vi "Package.vi"   [LabVIEW 2018, in "Scripts.lvlib"]
uses:
  Scripts.lvlib
  <vilib>/Field R&D Services/Labricator/Toolkit/Type Definitions/LabVIEW Versions.ctl
  <vilib>/Field R&D Services/Labricator/Toolkit/Field_RnD_Services_Labricator_Toolkit.lvlib
panel:
  # "Overview: Builds a VI Package (vip) for LabVIEW versions >= 2015\nRequirements: LabVIEW 2015, VIPM Pro, VIPM API, Labricator Development Kit, Labricator Run-Time\nInstructions: Run this VI.\n\nThis VI attempts to automate the building the VIP file for this add-on as much as possible. If VIPM Pro is not available, then the VIPM API will not work, and the building of the package must be done manually. This VI automates the following manual steps:\n\n1. Save the current project for LabVIEW 2015\n    a. From the Project Explorer window, select File>>Save for Previous Version... A new dialog will appear.\n    b. Select 15.0 from the drop down menu.\n    c. Click Save.... A new dialog will appear. Create a \"target\\15.0\" folder hierarchy in the root project folder (same location as the project file,    \n        .lvproj) if it does not already exist.\n    d. Click OK. All of the contents of the project will be saved to LabVIEW 2015.\n2. Copy the Help source to the target output\n    a. Start Windows Explorer.\n    b. Navigate to the \"<project root>\\src\" folder in Windows Explorer.\n    c. Copy the \"Help\" folder to the \"target\\15.0\\src\" location.\n3. Start LabVIEW 2015 and open the \"target\\15.0\\LIBSSH2.lvproj\" file created in Step 1. Do NOT open any file in the \"target\\15.0\" folder in any other \n    version of LabVIEW.\n4. Build all Source Distributions defined under \"Build Specifications\" tree item in the Project Explorer. A new \"target\\15.0\\builds\" folder will be \n    created with a sub-folder for each component.\n5. Expand the \"Configurations\" virtual folder in the Project Explorer and double click on the \"LabPack.vipb\" file. This will start the VIPM application.\n6. Click the \"Build\" icon near the top of the window for the LabPack package specification. Do NOT alter any values, but ensure \"2015\" is selected at \n    the top right.\n7. Once the package is built, it will be available at \"target\\15.0\\packages\".\n\nNote, any version newer than LabVIEW 2015 can be used to run this VI and still have the package built for LabVIEW 2015, but the LabVIEW 2015 development environment must be installed.\n\nWhen this VI runs, it will automatically start LabVIEW 2015, build all of the components, start VIPM, build the package, then close both LabVIEW 2015 and VIPM. Another VI, \"Build Target.vi\" will run during this process. Do not abort or close this VI while running."
types:
  T1 = typedef "Field_RnD_Services_Labricator_Toolkit.lvlib/LabVIEW Versions.ctl" = enum16{"2009", "2010", "2011", "2012", "2013", "2014", "2015", "2016", "2017", "2018"}
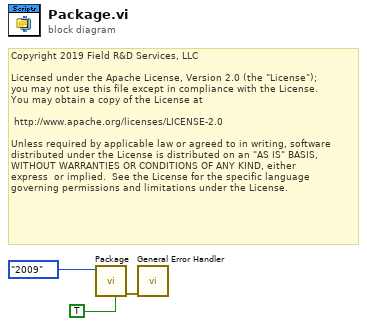
[diagram p0: block diagram]
diagram:
  # "Copyright 2019 Field R&D Services, LLC\n\nLicensed under the Apache License, Version 2.0 (the \"License\");\nyou may not use this file except in compliance with the License.\nYou may obtain a copy of the License at\n\n\thttp://www.apache.org/licenses/LICENSE-2.0\n\nUnless required by applicable law or agreed to in writing, software\ndistributed under the License is distributed on an \"AS IS\" BASIS,\nWITHOUT WARRANTIES OR CONDITIONS OF ANY KIND, either \nexpress  or implied.  See the License for the specific language \ngoverning permissions and limitations under the License."
  n1 = call <vilib>:"Package.vi"("Pre-Clean"=TRUE, "LabVIEW Previous Version"=LabVIEW_Versions."2009") -> ("Error Out"=w2:errorcluster)  [unwired: 9 in]
  n2 = call <vilib>:"General Error Handler.vi"("error in (no error)"=w2) -> ()  [unwired: 10 in, 5 out]
